vi "write general keywords.vi"(8 "error in (no error)":errorcluster, 11 "Save Image in":refnum<class "Save Image.lvclass">) -> (0 "error out":errorcluster, 3 "Save Image out":refnum<class "Save Image.lvclass">)   [LabVIEW 2018, in "Save Image.lvclass"]
uses:
  Save Image.lvclass
  Save Image.lvclass/Save Image.ctl
  Channel/Channel.lvclass/Channel.ctl
  Simulated_CCD_Camera/Simulated Camera.lvclass
  Channel/Channel.lvclass
panel:
  in  "Channel information":T1
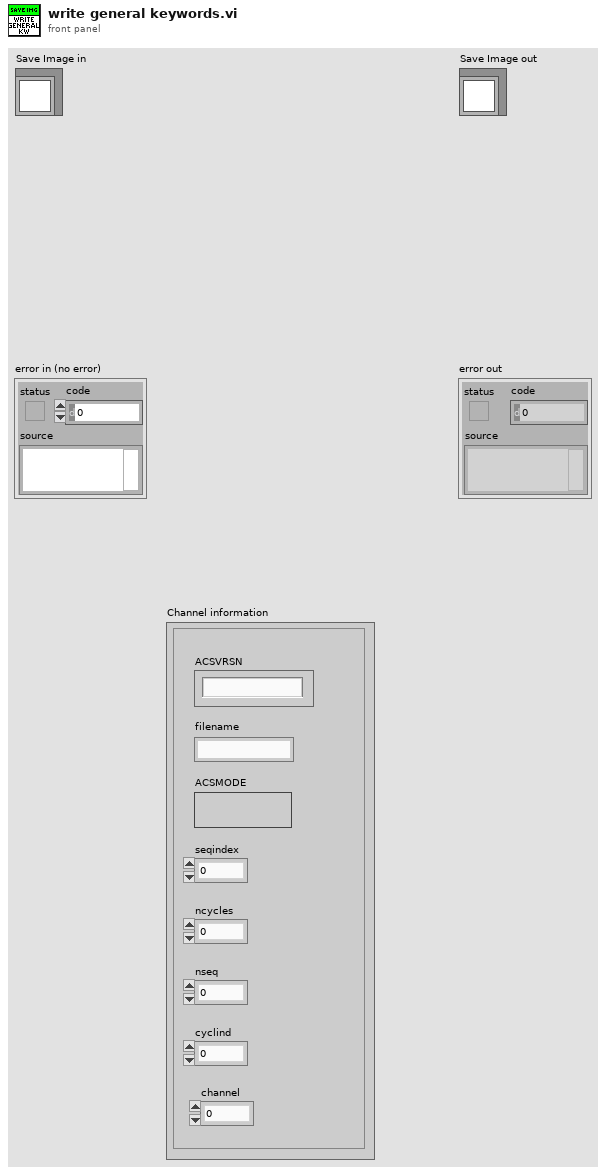
[diagram p1: front panel]
types:
  T1 = cluster{"ACSVRSN":string, "ACSMODE":bool, "filename":string, "seqindex":u16, "ncycles":u16, "nseq":u16, "cyclind":u16, "channel":u16}
  T2 = cluster{"Image path":path, "Remote IP":string, "Channel":u8, "ACS mode":u16, "Communication":u16}
  T3 = cluster{"CYCLES_DONE":u16, "LAST_IMAGE_NAME":string, "DISK_SPACE":u16, "FRAMES_DONE":u16, "CCD_STATUS":string, "CURRENT_TEMPERATURE":i16, "TEMPERATURE_STATUS":string, "FRAME_EXPOSURE_TIME":sgl, "ERROR":bool, "SERIAL_NUMBER":u16, "ACQUIRING":bool, "IMAGE_INDEX":u32, "SEQS_DONE":u16}
  T4 = cluster{"COOLER_POWER_STATUS":u16, "TEMP":i32, "EXPTIME":dbl, "#FRAMES":u32, "#CYCLES":u32, "#SEQS":u32, "WAVEPLATE_POS":u16}
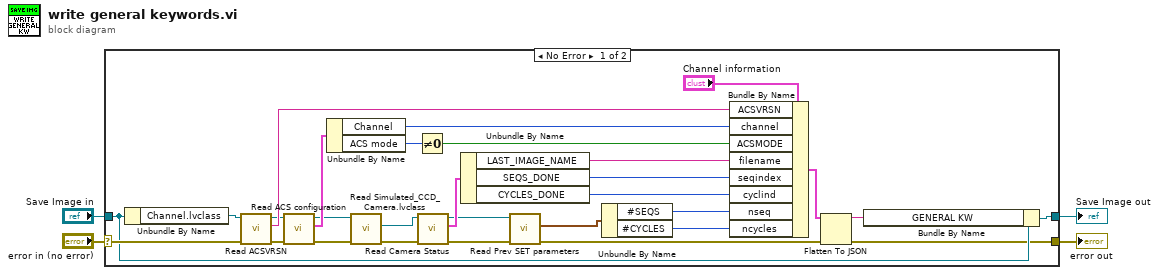
[diagram p0: block diagram]
diagram:
  n1 = case shown="No Error" "error in (no error)" {
    selector: "error in (no error)" -> [w30 w35]
    tunnel: [w13 w35] -> w3
    tunnel: [w10 w34] -> w1
    tunnel: "Save Image in" -> [w15 w34]
    frame No Error {
      n2 = Unbundle By Name(w15) -> ("Channel.lvclass"=w32:refnum<class "Channel.lvclass">)
      n3 = call "Read ACSVRSN.vi"("error in (no error)"=w30, "Channel in"=w32) -> ("error out"=w6:errorcluster, "ACSVRSN"=w31:string, "Channel out"=w7:refnum<class "Channel.lvclass">)  [unwired: 7 in]
      n4 = call-dynamic "Read ACS configuration.vi"("error in (no error)"=w6, "Channel in"=w7) -> ("error out"=w29:errorcluster, "acs init configuration"=w33:T2, "Channel out"=w28:refnum<class "Channel.lvclass">)  [unwired: 7 in]
      n5 = Unbundle By Name(w33) -> ("Channel"=w5:u8, "ACS mode"=w8:u16)
      n6 = call "Read Simulated_CCD_Camera.lvclass.vi"("error in (no error)"=w29, "Channel in"=w28) -> ("error out"=w26:errorcluster, "Simulated_CCD_Camera.lvclass"=w27:refnum<class "Simulated Camera.lvclass">)  [unwired: 7 in, 1 out]
      n7 = Not Equal To 0?(x=w8) -> (x != 0?=w9:bool)
      n8 = call "Read Camera Status.vi"("error in (no error)"=w26, "CCDCamera in"=w27) -> ("error out"=w25:errorcluster, "Camera Status"=w24:T3, "CCDCamera out"=w17:refnum<class "Simulated Camera.lvclass">)  [unwired: 7 in]
      n9 = Unbundle By Name(w24) -> ("LAST_IMAGE_NAME"=w23:string, "SEQS_DONE"=w22:u16, "CYCLES_DONE"=w21:u16)
      n10 = call-dynamic "Read Prev SET parameters.vi"("error in (no error)"=w25, "Simulated_CCD_Camera in"=w17) -> ("error out"=w14:errorcluster, "Prev SET parameters"=w20:T4)  [unwired: 7 in, 1 out]
      n11 = Unbundle By Name(w20) -> ("#SEQS"=w19:u32, "#CYCLES"=w18:u32)
      n12 = Bundle By Name(cluster="Channel information", "ACSVRSN"=w31, "channel"=w5, "ACSMODE"=w9, "filename"=w23, "seqindex"=w22, "cyclind"=w21, "nseq"=w19, "ncycles"=w18) -> (w11:T1)
      n13 = Flatten To JSON(anything=w11, error in (no error)=w14) -> (JSON string=w12:string, 11:w13:errorcluster)  [unwired: 1 in]
      n14 = Bundle By Name(cluster=w15, "GENERAL KW"=w12) -> (w10:refnum<class "Save Image.lvclass">)
    }
    frame Error {
    }
  }
  "error out" <- w3
  "Save Image out" <- w1
